vi "Liaison Série - 2 cam 2P.vi"(9 "timeout (ms)":u32=200, 11 "Port USB en réception":refnum<visa-resource-name>="ASRL1::INSTR") -> (0 "Indications pokaenmon D 2":T1, 1 "Indications pokaenmon G 2":T1, 2 "Indications pokaenmon D":T1, 3 "Indications pokaenmon G":T1, 4 "Nom VISA en sortie":refnum<visa-resource-name>)   [LabVIEW 2013]
uses:
  <vilib>/Instr/_visa.llb/VISA Configure Serial Port (Instr).vi
panel:
  out "error out":errorcluster caption="sortie d'erreur"
  out "Sortie lue":string
  # "Réception de données-XBee"
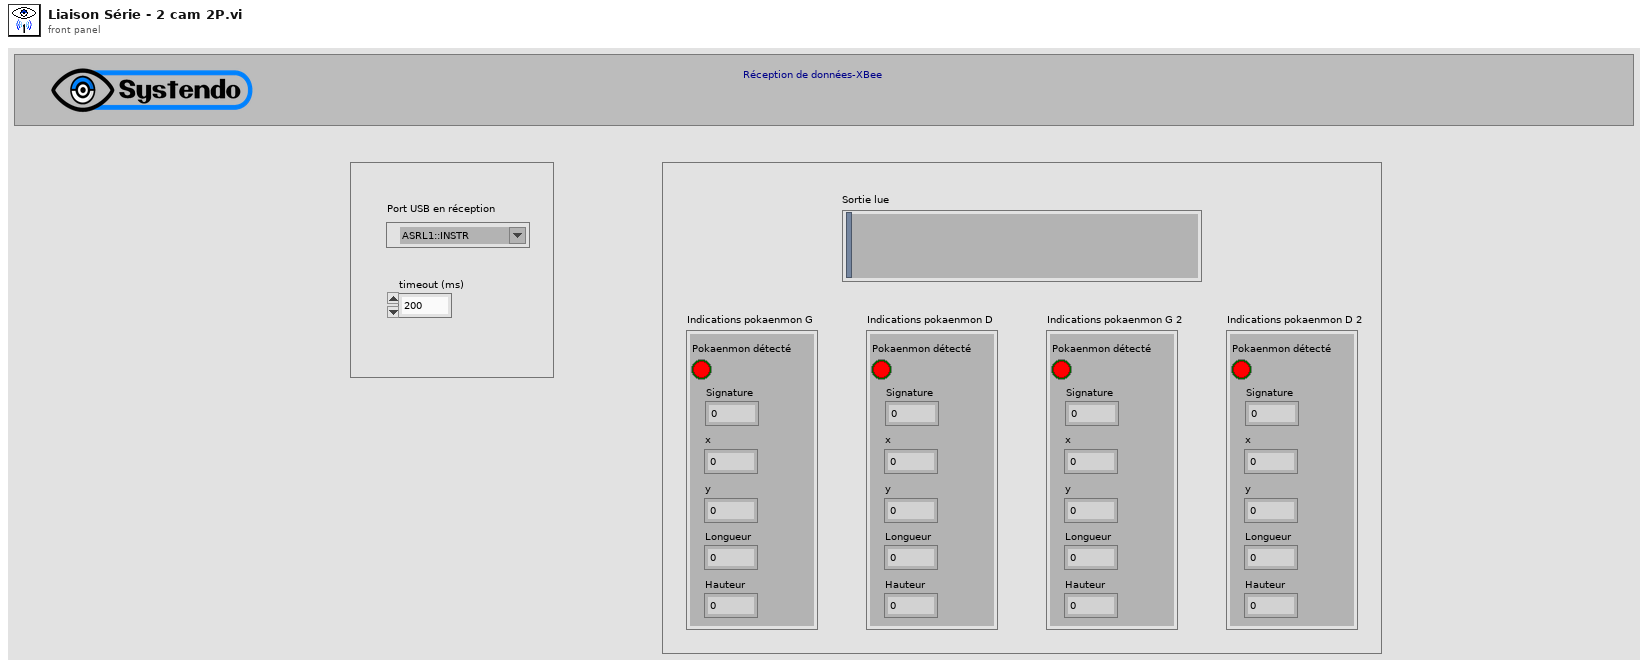
[diagram p1: front panel]
types:
  T1 = cluster{"Pokaenmon détecté":bool, "Signature":u32, "x":dbl, "y ":dbl, "Longueur":dbl, "Hauteur":dbl}
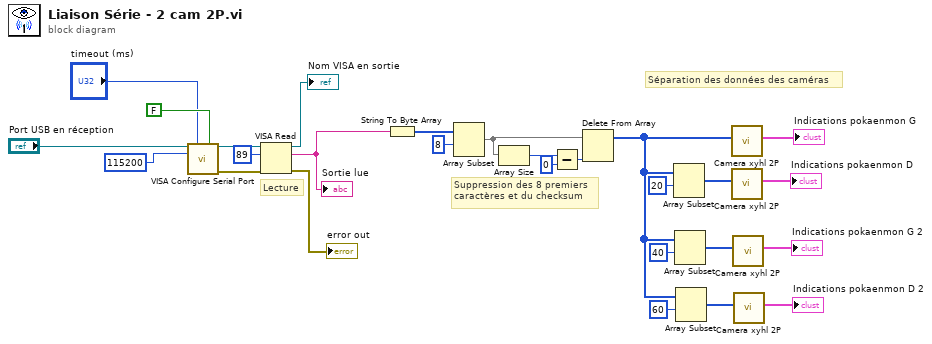
[diagram p0: block diagram]
diagram:
  # "Séparation des données des caméras"
  # "Suppression des 8 premiers\ncaractères et du checksum"
  # "Lecture"
  n1 = call-poly "VISA Configure Serial Port"("VISA resource name"="Port USB en réception", "timeout (10sec)"="timeout (ms)", "Enable Termination\nChar (T)"=FALSE ("Enable Termination\nChar (T)"), "baud rate (9600)"=u32 115200 ("Baud Rate (115200)")) -> ("VISA resource name out"=w17:refnum<visa-resource-name>, "error out"=w15:errorcluster)  [unwired: 10 in]
  n2 = VISA Read(VISA resource name=w17, byte count=u32 89 ("nombre d'octets"), error in (no error)=w15) -> (VISA resource name out=→"Nom VISA en sortie":refnum<visa-resource-name>, read buffer=w27:string, error out=→"error out":errorcluster)  [unwired: 1 out]
  "Sortie lue" <- w27
  n3 = String To Byte Array(string=w27) -> (unsigned byte array=w24:u8[])
  n4 = Array Subset(array=w24, index=8 ("offset (0)")) -> (w13:u8[])  [unwired: 1 in]
  n5 = Array Size(array=w13) -> (size(s)=w25:i32)
  n6 = Subtract(x=w25, y=0) -> (x-y=w26:i32)
  n7 = Delete From Array(array=w13, index=w26) -> (array with subset deleted=w1:u8[])  [unwired: 1 in, 1 out]
  n8 = Array Subset(array=w1, index=20 ("indice")) -> (w10:u8[])  [unwired: 1 in]
  n9 = Array Subset(array=w1, index=40 ("indice")) -> (w6:u8[])  [unwired: 1 in]
  n10 = Array Subset(array=w1, index=60 ("indice")) -> (w3:u8[])  [unwired: 1 in]
  n11 = call "Camera xyhl 2P.vi"("tableau"=w1) -> ("Indications pokaenmon"=→"Indications pokaenmon G":T1)  [unwired: 10 in]
  n12 = call "Camera xyhl 2P.vi"("tableau"=w10) -> ("Indications pokaenmon"=→"Indications pokaenmon D":T1)  [unwired: 10 in]
  n13 = call "Camera xyhl 2P.vi"("tableau"=w6) -> ("Indications pokaenmon"=→"Indications pokaenmon G 2":T1)  [unwired: 10 in]
  n14 = call "Camera xyhl 2P.vi"("tableau"=w3) -> ("Indications pokaenmon"=→"Indications pokaenmon D 2":T1)  [unwired: 10 in]
